vi "PS Control Run v0.80.vi"(2 "error in (no error)":errorcluster) -> (0 "error out":errorcluster, 1 "Time(ms)":u32)   [LabVIEW 2020]
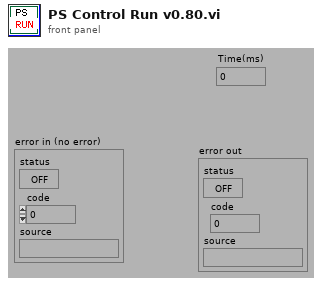
[diagram p1: front panel]
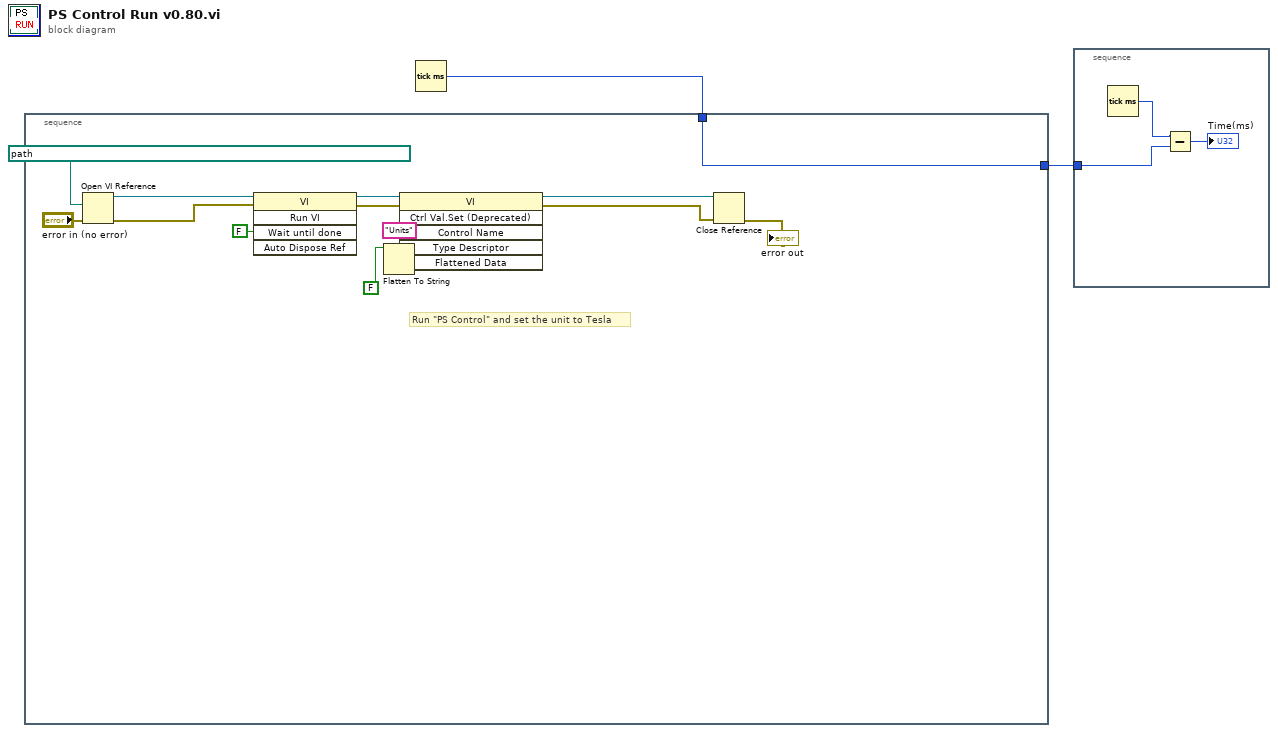
[diagram p0: block diagram]
diagram:
  n1 = Tick Count (ms)() -> (millisecond timer value=w2:u32)
  n2 = stacked-sequence {
    tunnel: [w16] -> w1
    tunnel: w2 -> [w16]
    frame #0 {
      # "Run \"PS Control\" and set the unit to Tesla"
      n3 = Open VI Reference(vi path=path "/Optics2Mac/xwei Work/NML Data Acq/Serial Instruments/PS Ä/PS Control", error in (no error)="error in (no error)") -> (vi reference=w15:refnum<vi>, error out=w13:errorcluster)  [unwired: 4 in]
      n4 = invoke class="VI" method="Run VI"(reference=w15, error in=w13, "Wait until done"=FALSE) -> (reference out=w6:refnum<vi>, error out=w4:errorcluster)  [unwired: 2 in, 3 out]
      n5 = Flatten To String(anything=FALSE ("Wait until done")) -> (data string=w10:string, type string=w9:i16[])  [unwired: 3 in, 1 out]
      n6 = invoke class="VI" method="Ctrl Val.Set (Deprecated)"(reference=w6, error in=w4, "Control Name"="Units", "Type Descriptor"=w9, "Flattened Data"=w10) -> (reference out=w5:refnum<vi>, error out=w3:errorcluster)  [unwired: 1 in, 4 out]
      n7 = Close Reference(reference=w5, error in (no error)=w3) -> (error out=→"error out":errorcluster)
    }
  }
  n8 = stacked-sequence {
    tunnel: w1 -> [w19]
    frame #0 {
      n9 = Tick Count (ms)() -> (millisecond timer value=w20:u32)
      n10 = Subtract(x=w20, y=w19) -> (x-y=→"Time(ms)":u32)
    }
  }
